vi "Set ManualAO.vi"(8 "error in":errorcluster, 9 "Manual Output Value (0.000)":dbl min=0.0 max=20.0 step=0.001 format="%.3f", 10 "Channel (0001)":string="0001", 11 "VISA resource name":refnum<visa-resource-name>) -> (0 "error out":errorcluster, 2 "Channel":string, 3 "VISA resource name out":refnum<visa-resource-name>)   [LabVIEW 2020, in "Yokogawa GX Series.lvlib"]
doc: "This VI sets manual output AO channel."
uses:
  <instrlib>/Yokogawa GX Series/Yokogawa GX Series.lvlib
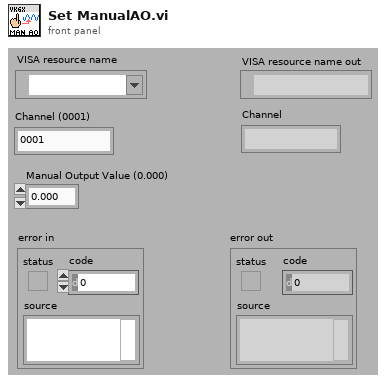
[diagram p1: front panel]
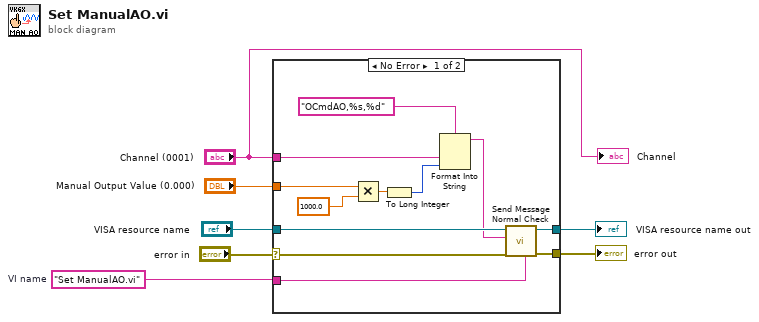
[diagram p0: block diagram]
diagram:
  w7 = "Set ManualAO.vi"  # VI name
  n1 = case shown="No Error" "error in" {
    selector: "error in" -> [w10 w21]
    tunnel: [w8 w20] -> w4
    tunnel: [w19 w21] -> w1
    tunnel: w7 -> [w9 _]
    tunnel: "Channel (0001)" -> [w18 _]
    tunnel: "Manual Output Value (0.000)" -> [w16 _]
    tunnel: "VISA resource name" -> [w12 w20]
    frame No Error {
      n2 = Multiply(x=w16, y=1000.0) -> (x*y=w14:dbl)
      n3 = To Long Integer(number=w14) -> (32bit integer=w13:i32)
      n4 = Format Into String(format string="OCmdAO,%s,%d", w18, w13) -> (resulting string=w11:string)  [unwired: 2 in, 1 out]
      n5 = call <instrlib>:"Send Message Normal Check.vi"("Source (\"\")"=w9, "error in (no error)"=w10, "Send Message (\"\")"=w11, "VISA resource name"=w12) -> ("error out"=w19:errorcluster, "VISA resource name out"=w8:refnum<visa-resource-name>)  [unwired: 2 in, 4 out]
    }
    frame Error {
    }
  }
  "VISA resource name out" <- w4
  "error out" <- w1
  "Channel" <- "Channel (0001)"
